vi "Init & Start Sequence.vi"(8 "error in (no error)":errorcluster, 9 "Channel Mask":u64, 10 "Config Data":T2, 11 "Connection Data In":T1) -> (0 "error out":errorcluster, 3 "Connection Data Out":T1)   [LabVIEW 2014, in "MSX-E3711_dll.lvlib"]
doc: "Toma los datos de configuracion y su dll se encarga de pasarle los parametros al ADDI-DATA."
uses:
  MSX-E3711_dll.lvlib
  Typedef/Config Data.ctl
  Typedef/Connection Data.ctl
  E:/Repositorio Magnis/INF002/v0/Modules/HAL/Drivers/Sync/ADDI-DATA MSX-E3711/API/MSXE371x.dll
  MSXE371x.dll
  E:/Repositorio Magnis/INF002/v0/Modules/HAL/Drivers/Sync/ADDI-DATA MSX-E3711/API/MXCommon.dll
  MXCommon.dll
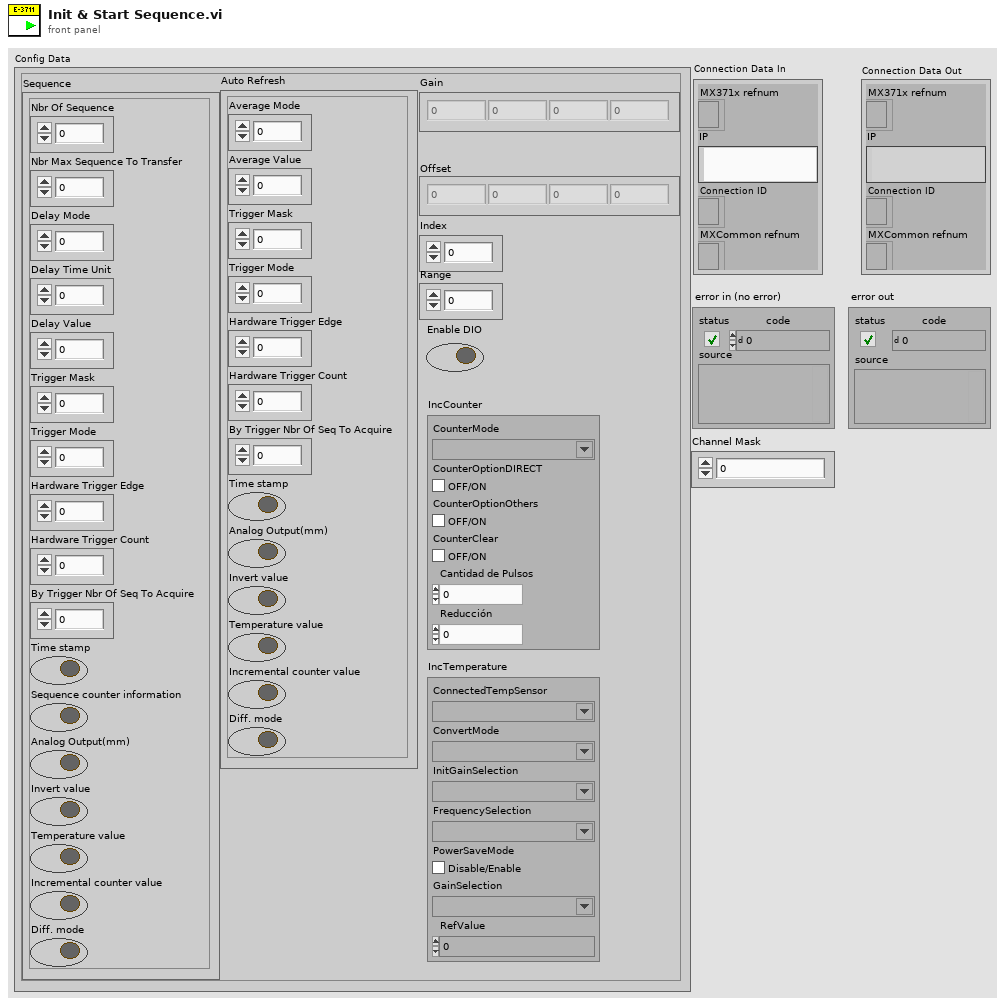
[diagram p1: front panel]
types:
  T1 = typedef "MSX-E3711_dll.lvlib/Connection Data.ctl" = cluster{"MX371x refnum":refnum<k24>, "IP":string, "Connection ID ":refnum<k5>, "MXCommon refnum":refnum<k24>}
  T2 = typedef "MSX-E3711_dll.lvlib/Config Data.ctl" = cluster{"Auto Refresh":cluster{"Average Mode":u64, "Average Value":u64, "Trigger Mask":u64, "Trigger Mode":u64, "Hardware Trigger Edge":u64, "Hardware Trigger Count":u64, "By Trigger Nbr Of Seq To Acquire":u64, "Time stamp":bool, "Analog Output(mm)":bool, "Invert value":bool, "Temperature value":bool, "Incremental counter value":bool, "Diff. mode":bool}, "Gain":sgl[], "Offset":sgl[], "Index":u64, "Range":sgl, "Sequence":cluster{"Nbr Of Sequence":u64, "Nbr Max Sequence To Transfer":u64, "Delay Mode":u64, "Delay Time Unit":u64, "Delay Value":u64, "Trigger Mask":u64, "Trigger Mode":u64, "Hardware Trigger Edge":u64, "Hardware Trigger Count":u64, "By Trigger Nbr Of Seq To Acquire":u64, "Time stamp":bool, "Sequence counter information":bool, "Analog Output(mm)":bool, "Invert value":bool, "Temperature value":bool, "Incremental counter value":bool, "Diff. mode":bool}, "Enable DIO":bool, "IncCounter":cluster{"CounterMode":string, "CounterOptionDIRECT  ":bool, "CounterOptionOthers":bool, "CounterClear ":bool, "Cantidad de Pulsos":sgl, "Reducción":sgl}, "IncTemperature":cluster{"ConnectedTempSensor":string, "ConvertMode":string, "InitGainSelection":string, "FrequencySelection":string, "PowerSaveMode":bool, "GainSelection":string, "RefValue":dbl}}
  T3 = cluster{"Nbr Of Sequence":u64, "Nbr Max Sequence To Transfer":u64, "Delay Mode":u64, "Delay Time Unit":u64, "Delay Value":u64, "Trigger Mask":u64, "Trigger Mode":u64, "Hardware Trigger Edge":u64, "Hardware Trigger Count":u64, "By Trigger Nbr Of Seq To Acquire":u64, "Time stamp":bool, "Sequence counter information":bool, "Analog Output(mm)":bool, "Invert value":bool, "Temperature value":bool, "Incremental counter value":bool, "Diff. mode":bool}
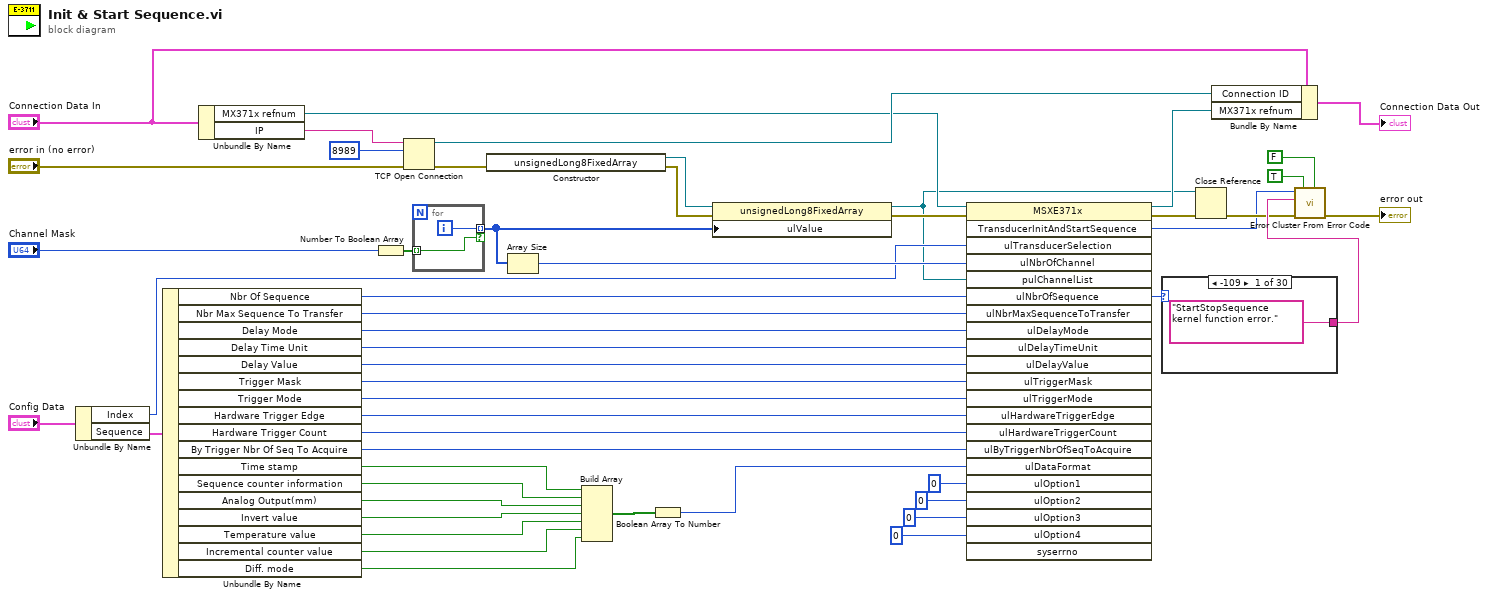
[diagram p0: block diagram]
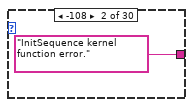
[diagram p2: hidden frame]
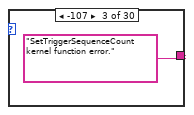
[diagram p3: hidden frame]
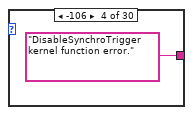
[diagram p4: hidden frame]
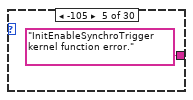
[diagram p5: hidden frame]
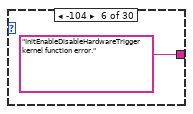
[diagram p6: hidden frame]
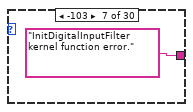
[diagram p7: hidden frame]
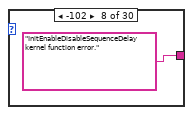
[diagram p8: hidden frame]
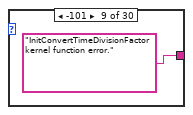
[diagram p9: hidden frame]
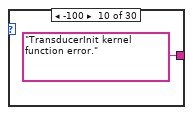
[diagram p10: hidden frame]
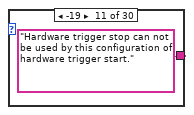
[diagram p11: hidden frame]
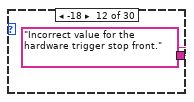
[diagram p12: hidden frame]
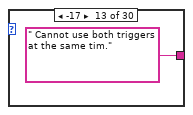
[diagram p13: hidden frame]
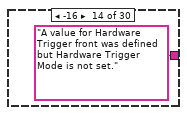
[diagram p14: hidden frame]
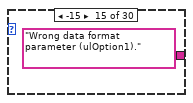
[diagram p15: hidden frame]
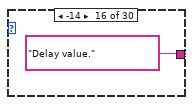
[diagram p16: hidden frame]
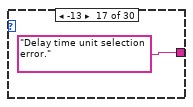
[diagram p17: hidden frame]
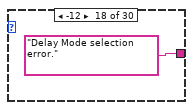
[diagram p18: hidden frame]
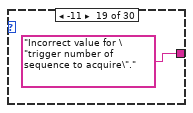
[diagram p19: hidden frame]
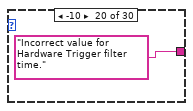
[diagram p20: hidden frame]
diagram:
  n1 = Unbundle By Name("Config Data") -> ("Index"=w25:u64, "Sequence"=w49:T3)
  n2 = Unbundle By Name(w49) -> ("Nbr Of Sequence"=w24:u64, "Nbr Max Sequence To Transfer"=w23:u64, "Delay Mode"=w22:u64, "Delay Time Unit"=w21:u64, "Delay Value"=w20:u64, "Trigger Mask"=w19:u64, "Trigger Mode"=w18:u64, "Hardware Trigger Edge"=w17:u64, "Hardware Trigger Count"=w16:u64, "By Trigger Nbr Of Seq To Acquire"=w15:u64, "Time stamp"=w47:bool, "Sequence counter information"=w42:bool, "Analog Output(mm)"=w43:bool, "Invert value"=w44:bool, "Temperature value"=w45:bool, "Incremental counter value"=w46:bool, "Diff. mode"=w1:bool)
  n3 = Unbundle By Name("Connection Data In") -> ("MX371x refnum"=w27:refnum<k24>, "IP"=w32:string)
  n4 = Number To Boolean Array(number="Channel Mask") -> (Boolean array=w50:bool[])
  n5 = TCP Open Connection(address=w32, remote port or service name=u16 8989 ("Netzwerk-Port"), error in (no error)="error in (no error)") -> (connection ID=w33:refnum<k5>, error out=w9:errorcluster)  [unwired: 2 in]
  n6 = for {
    tunnel: [w52] -> w4 mode=indexing if=w51
    tunnel: w50 -> [w51] mode=indexing
    i -> [w52]
  }
  n7 = constructor class="unsignedLong8FixedArray"(error in=w9) -> (reference out=w8:refnum<k24>, error out=w7:errorcluster)  [unwired: 2 in, 1 out]
  n8 = Array Size(array=w4) -> (size(s)=w26:i32)
  n9 = Build Array(w47, w42, w43, w44, w45, w46, w1) -> (w48:bool[])
  n10 = Boolean Array To Number(Boolean array=w48) -> (number=w14:u32)
  n11 = property class="unsignedLong8FixedArray"(reference=w8, error in=w7, "ulValue"=w4) -> (reference out=w5:refnum<k24>, error out=w6:errorcluster)
  n12 = invoke class="MSXE371x" method="TransducerInitAndStartSequence"(reference=w27, error in=w6, "ulTransducerSelection"=w25, "ulNbrOfChannel"=w26, "pulChannelList"=w5, "ulNbrOfSequence"=w24, "ulNbrMaxSequenceToTransfer"=w23, "ulDelayMode"=w22, "ulDelayTimeUnit"=w21, "ulDelayValue"=w20, "ulTriggerMask"=w19, "ulTriggerMode"=w18, "ulHardwareTriggerEdge"=w17, "ulHardwareTriggerCount"=w16, "ulByTriggerNbrOfSeqToAcquire"=w15, "ulDataFormat"=w14, "ulOption1"=u64 0 ("ulOption2"), "ulOption2"=u64 0 ("ulOption3"), "ulOption3"=u64 0 ("ulOption4"), "ulOption4"=u64 0) -> (reference out=w30:refnum<k24>, error out=w29:errorcluster, "TransducerInitAndStartSequence"=w28:i32)  [unwired: 2 in, 19 out]
  n13 = case shown="-109" w28 {
    tunnel: ["StartStopSequence kernel function error." "InitSequence kernel function error." "SetTriggerSequenceCount kernel function error." "DisableSynchroTrigger kernel function error." "InitEnableSynchroTrigger kernel function error." "InitEnableDisableHardwareTrigger kernel function error." "InitDigitalInputFilter kernel function error." "InitEnableDisableSequenceDelay kernel function error." "InitConvertTimeDivisionFactor kernel function error." "TransducerInit kernel function error." "Hardware trigger stop can not be used by this configuration of hardware trigger start." "Incorrect value for the hardware trigger stop front." " Cannot use both triggers at the same tim." "A value for Hardware Trigger front was defined but Hardware Trigger Mode is not set." "Wrong data format parameter (ulOption1)." "Delay value." "Delay time unit selection error." "Delay Mode selection error." "Incorrect value for \"trigger number of sequence to acquire\"." "Incorrect value for Hardware Trigger filter time." "Incorrect value for Hardware Trigger Count." "Incorrect value for Synchro Trigger Mode." "Incorrect value for Hardware Trigger Front." "Incorrect value for Hardware Trigger Mode." "Division factor error." "Channel array selection error." "Number of channel error." "Transducer selection error." "Means an system error occurred." "Success."] -> w39
    frame -109 {
    }
    frame -108 {
    }
    frame -107 {
    }
    frame -106 {
    }
    frame -105 {
    }
    frame -104 {
    }
    frame -103 {
    }
    frame -102 {
    }
    frame -101 {
    }
    frame -100 {
    }
    frame -19 {
    }
    frame -18 {
    }
    frame -17 {
    }
    frame -16 {
    }
    frame -15 {
    }
    frame -14 {
    }
    frame -13 {
    }
    frame -12 {
    }
    frame -11 {
    }
    frame -10 {
    }
    frame -9 {
    }
    frame -8 {
    }
    frame -7 {
    }
    frame -6 {
    }
    frame -5 {
    }
    frame -4 {
    }
    frame -3 {
    }
    frame -2 {
    }
    frame -1 {
    }
    frame 0, Default {
    }
  }
  n14 = Close Reference(reference=w5, error in (no error)=w29) -> (error out=w38:errorcluster)
  n15 = Bundle By Name(cluster="Connection Data In", "Connection ID"=w33, "MX371x refnum"=w30) -> (→"Connection Data Out":T1)
  n16 = call <vilib>:"Error Cluster From Error Code.vi"("is warning? (False)"=FALSE, "show call chain? (False)"=TRUE, "error in (no error)"=w38, "error message (\"\")"=w39, "error code (0)"=w28) -> ("error out"=→"error out":errorcluster)  [unwired: 4 in]
